vi "SN_Data.vi"(10 "type":i32, 11 "String":string) -> (2 "Array":T1(array[cluster]))   [LabVIEW 2017]
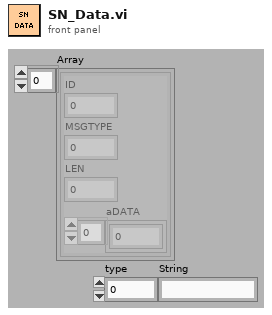
[diagram p1: front panel]
types:
  T1 = cluster{"ID":u32, "MSGTYPE":u8, "LEN":u8, "aDATA":u8[]}[]
  T2 = cluster{"ID":u32, "MSGTYPE":u8, "LEN":u8, "aDATA":u8[]}
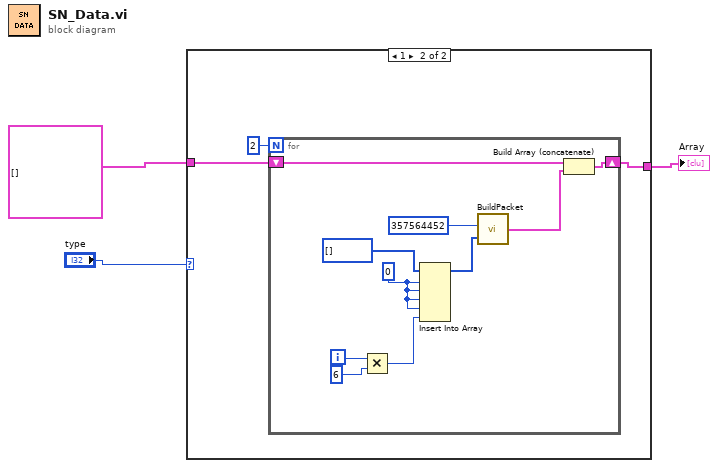
[diagram p0: block diagram]
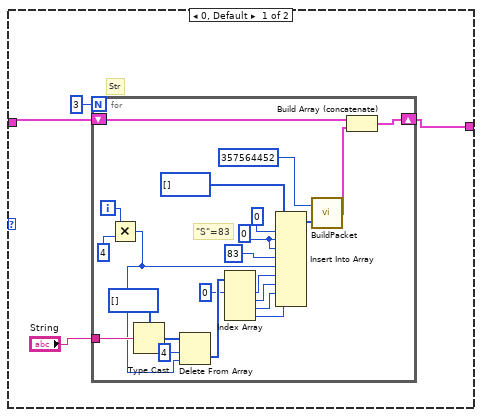
[diagram p2: hidden frame]
diagram:
  n1 = case shown="1" "type" {
    tunnel: T1 [] ("Array") -> [w6 w32]
    tunnel: [w5 w31] -> w2
    frame 0, Default {
      # "Str"
      n2 = for {
        N: 3 -> [_]
        shift-right: [w23] -> w5
        shift-left: w6 -> [w29]
        tunnel: "String" -> [w12]
        i -> [w10]
        w9 = 0 ("index")
        # "\"S\"=83"
        n3 = Multiply(x=w10, y=4) -> (x*y=w8:i32)
        n4 = Type Cast(type=u8[] [], x=w12) -> (*(type *) &x=w20:u8[])
        n5 = Delete From Array(array=w20, length=4, index=w8) -> (deleted portion=w22:u8[])  [unwired: 1 out]
        n6 = Index Array(array=w22, index #1=0 ("index")) -> (element #1=w17:u8, element #2=w16:u8, element #3=w15:u8, element #4=w14:u8)  [unwired: 3 in]
        n7 = Insert Into Array(array=u8[] [] ("Data 2"), index=0, new element #1=w9, new element #2=w9, new element #3=u8 83 ("new element/subarray"), new element #4=w8, new element #5=w17, new element #6=w16, new element #7=w15, new element #8=w14) -> (w26:u8[])
        n8 = call "BuildPacket.vi"("Data"=w26, "TxID"=u32 357564452 ("Param ID")) -> ("MsgTX 2"=w28:T2)
        n9 = Build Array (concatenate)(w29, w28) -> (w23:T1)
      }
    }
    frame 1 {
      n10 = for {
        N: 2 -> [_]
        shift-right: [w40] -> w31
        shift-left: w32 -> [w42]
        i -> [w36]
        w33 = 0 ("index")
        n11 = Multiply(x=w36, y=6) -> (x*y=w34:i32)
        n12 = Insert Into Array(array=u8[] [] ("Data 2"), index=w33, new element #1=w33, new element #2=w33, new element #3=w33, new element #4=w34) -> (w38:u8[])
        n13 = call "BuildPacket.vi"("Data"=w38, "TxID"=u32 357564452) -> ("MsgTX 2"=w41:T2)
        n14 = Build Array (concatenate)(w42, w41) -> (w40:T1)
      }
    }
  }
  "Array" <- w2
